vi "LV SciSDK FFT ARM.vi"(8 "error in (no error)":errorcluster, 9 "Board Handle In":T1, 10 "FFT Handle In":cluster{"FFT Path":string, "FFT Name":string}) -> (0 "error out":errorcluster, 1 "Board Handle Out":T1, 2 "FFT Handle Out":cluster{"FFT Path":string, "FFT Name":string}, 3 "NI Error Code":i32)   [LabVIEW 2021]
uses:
  SciSDK_Labview.lvlib
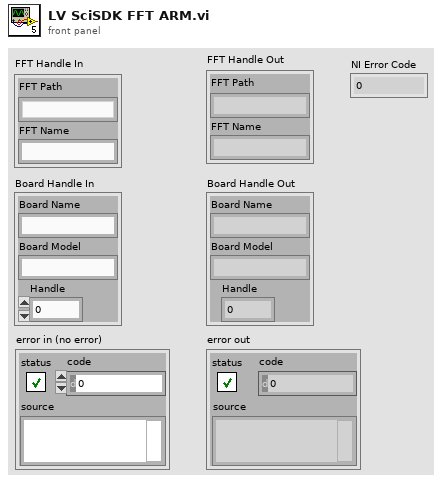
[diagram p1: front panel]
types:
  T1 = cluster{"Board Name":string, "Board Model":string, "Handle":u64}
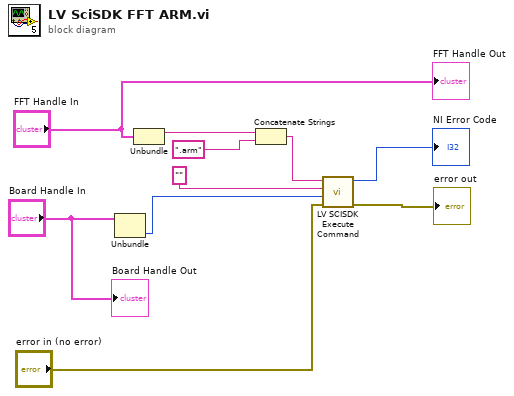
[diagram p0: block diagram]
diagram:
  n1 = Unbundle("Board Handle In") -> ("Handle"=w3:u64)  [unwired: 2 out]
  n2 = Unbundle("FFT Handle In") -> ("FFT Path"=w4:string)  [unwired: 1 out]
  n3 = Concatenate Strings(w4, ".arm" ("string")) -> (w8:string)
  n4 = call "LV SCISDK Execute Command.vi"("error in (no error)"="error in (no error)", "handle"=w3, "value"="", "Path"=w8) -> ("error out"=→"error out":errorcluster, "function return"=→"NI Error Code":i32)  [unwired: 5 in, 1 out]
  "FFT Handle Out" <- "FFT Handle In"
  "Board Handle Out" <- "Board Handle In"
